vi "ExtendedKalmanFilter_New.vi"(5 "States":i32, 6 "Extended_KALMAN_FUNC_GROUP":T1, 7 "Inputs":i32, 8 "dt_Seconds":dbl=0.02, 9 "MeasurementStdDevs":T3, 10 "StateStdDevs":T3, 11 "Outputs":i32) -> (0 "Error":bool, 3 "ExtendedKalmanFiilter":T4)   [LabVIEW 2019, in "Trajectory_Library.lvlib"]
doc: "Kalman filters combine predictions from a model and measurements to give an estimate of the true system state. This is useful because many states cannot be measured directly as a result of sensor noise, or because the state is \"hidden\".\n \nThe Extended Kalman filter is just like the KalmanFilter Kalman filter, but we make a linear approximation of nonlinear dynamics and/or nonlinear measurement models. This means that the EKF works with nonlinear systems.\n\nConstructs an extended Kalman filter.\n \n - states -- the number of states.\n - inputs -- the number of inputs.\n - outputs -- the number of outputs.\n - ExtendedKalmanFuncGroup -- definition of external functions used by this filter. it includes:\n - f_func -- A vector-valued function of x and u that returns the derivative of the state vector.\n - f_FuncExtra -- extra data, if any, used by the F_Func\n - h_func -- A vector-valued function of x and u that returns the measurement vector.\n - h_FuncExtra -- extra data, if any, used by the H_Func\n - stateStdDevs -- Standard deviations of model states.\n - measurementStdDevs -- Standard deviations of measurements.\n - dtSeconds -- Nominal discretization timestep.\n\nOutputs:\n - ExtendedKalmanFilter -- filter data cluster"
uses:
  Trajectory_Library.lvlib
  <vilib>/Analysis/Matrix/Datatypes/RealMatrix.ctl
  <vilib>/Analysis/Matrix/NI_Matrix.lvlib
  TypeDef/EXTENDED_KALMAN_FILTER.ctl
  <vilib>/Analysis/NI_AALPro.lvlib
  <vilib>/Analysis/7linalg.llb/Real Transpose Matrix.vi
  TypeDef/CALLBACK_FUNC_TYPE.ctl
  TypeDef/EXTENDED_KALMAN_CORRECT_FUNC_GROUP.ctl
panel:
  # "<States,1>"
  # "<Outputs,1>"
  # "State Estimate <Statess,1>"
  # "<States, States>"
  # "<States, States>"
  # "<Statess,  States>"
  # "<Outputs, Outputs>"
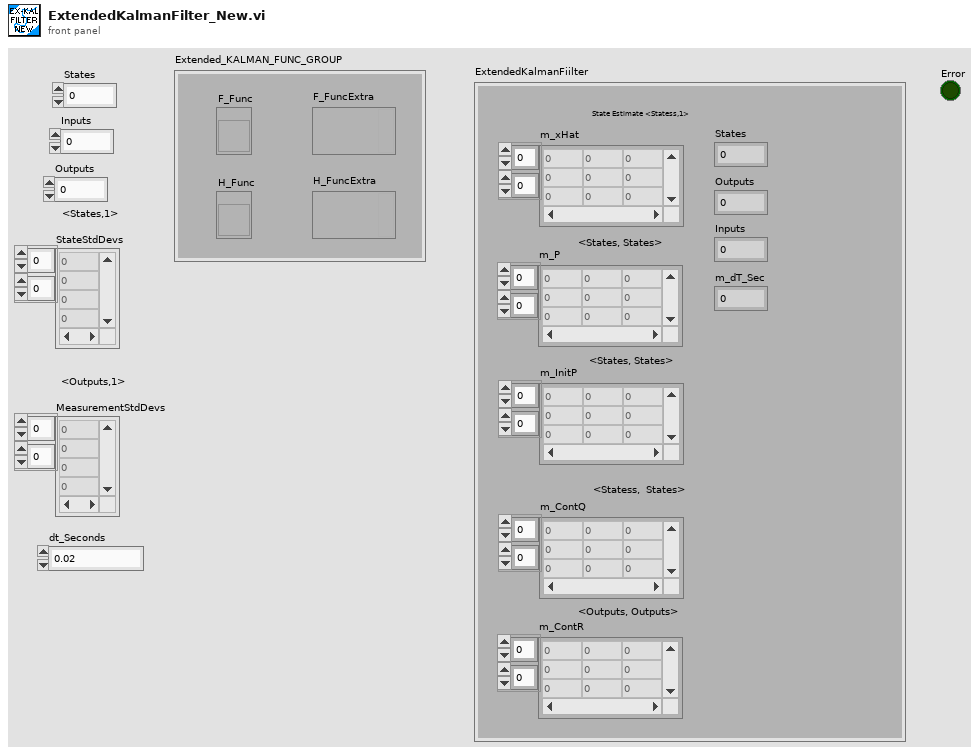
[diagram p1: front panel]
types:
  T1 = typedef "Trajectory_Library.lvlib/EXTENDED_KALMAN_CORRECT_FUNC_GROUP.ctl" = cluster{"H_Func":T2, "F_Func":T2, "H_FuncExtra":variant, "F_FuncExtra":variant}
  T2 = typedef "Trajectory_Library.lvlib/CALLBACK_FUNC_TYPE.ctl" = refnum<vi>
  T3 = typedef "NI_Matrix.lvlib/RealMatrix.ctl" = dbl[][]
  T4 = typedef "Trajectory_Library.lvlib/EXTENDED_KALMAN_FILTER.ctl" = cluster{"m_P":T3, "m_xHat":T3, "States":i32, "Outputs":i32, "m_ContR":T3, "m_ContQ":T3, "m_dT_Sec":dbl, "Inputs":i32, "m_InitP":T3}
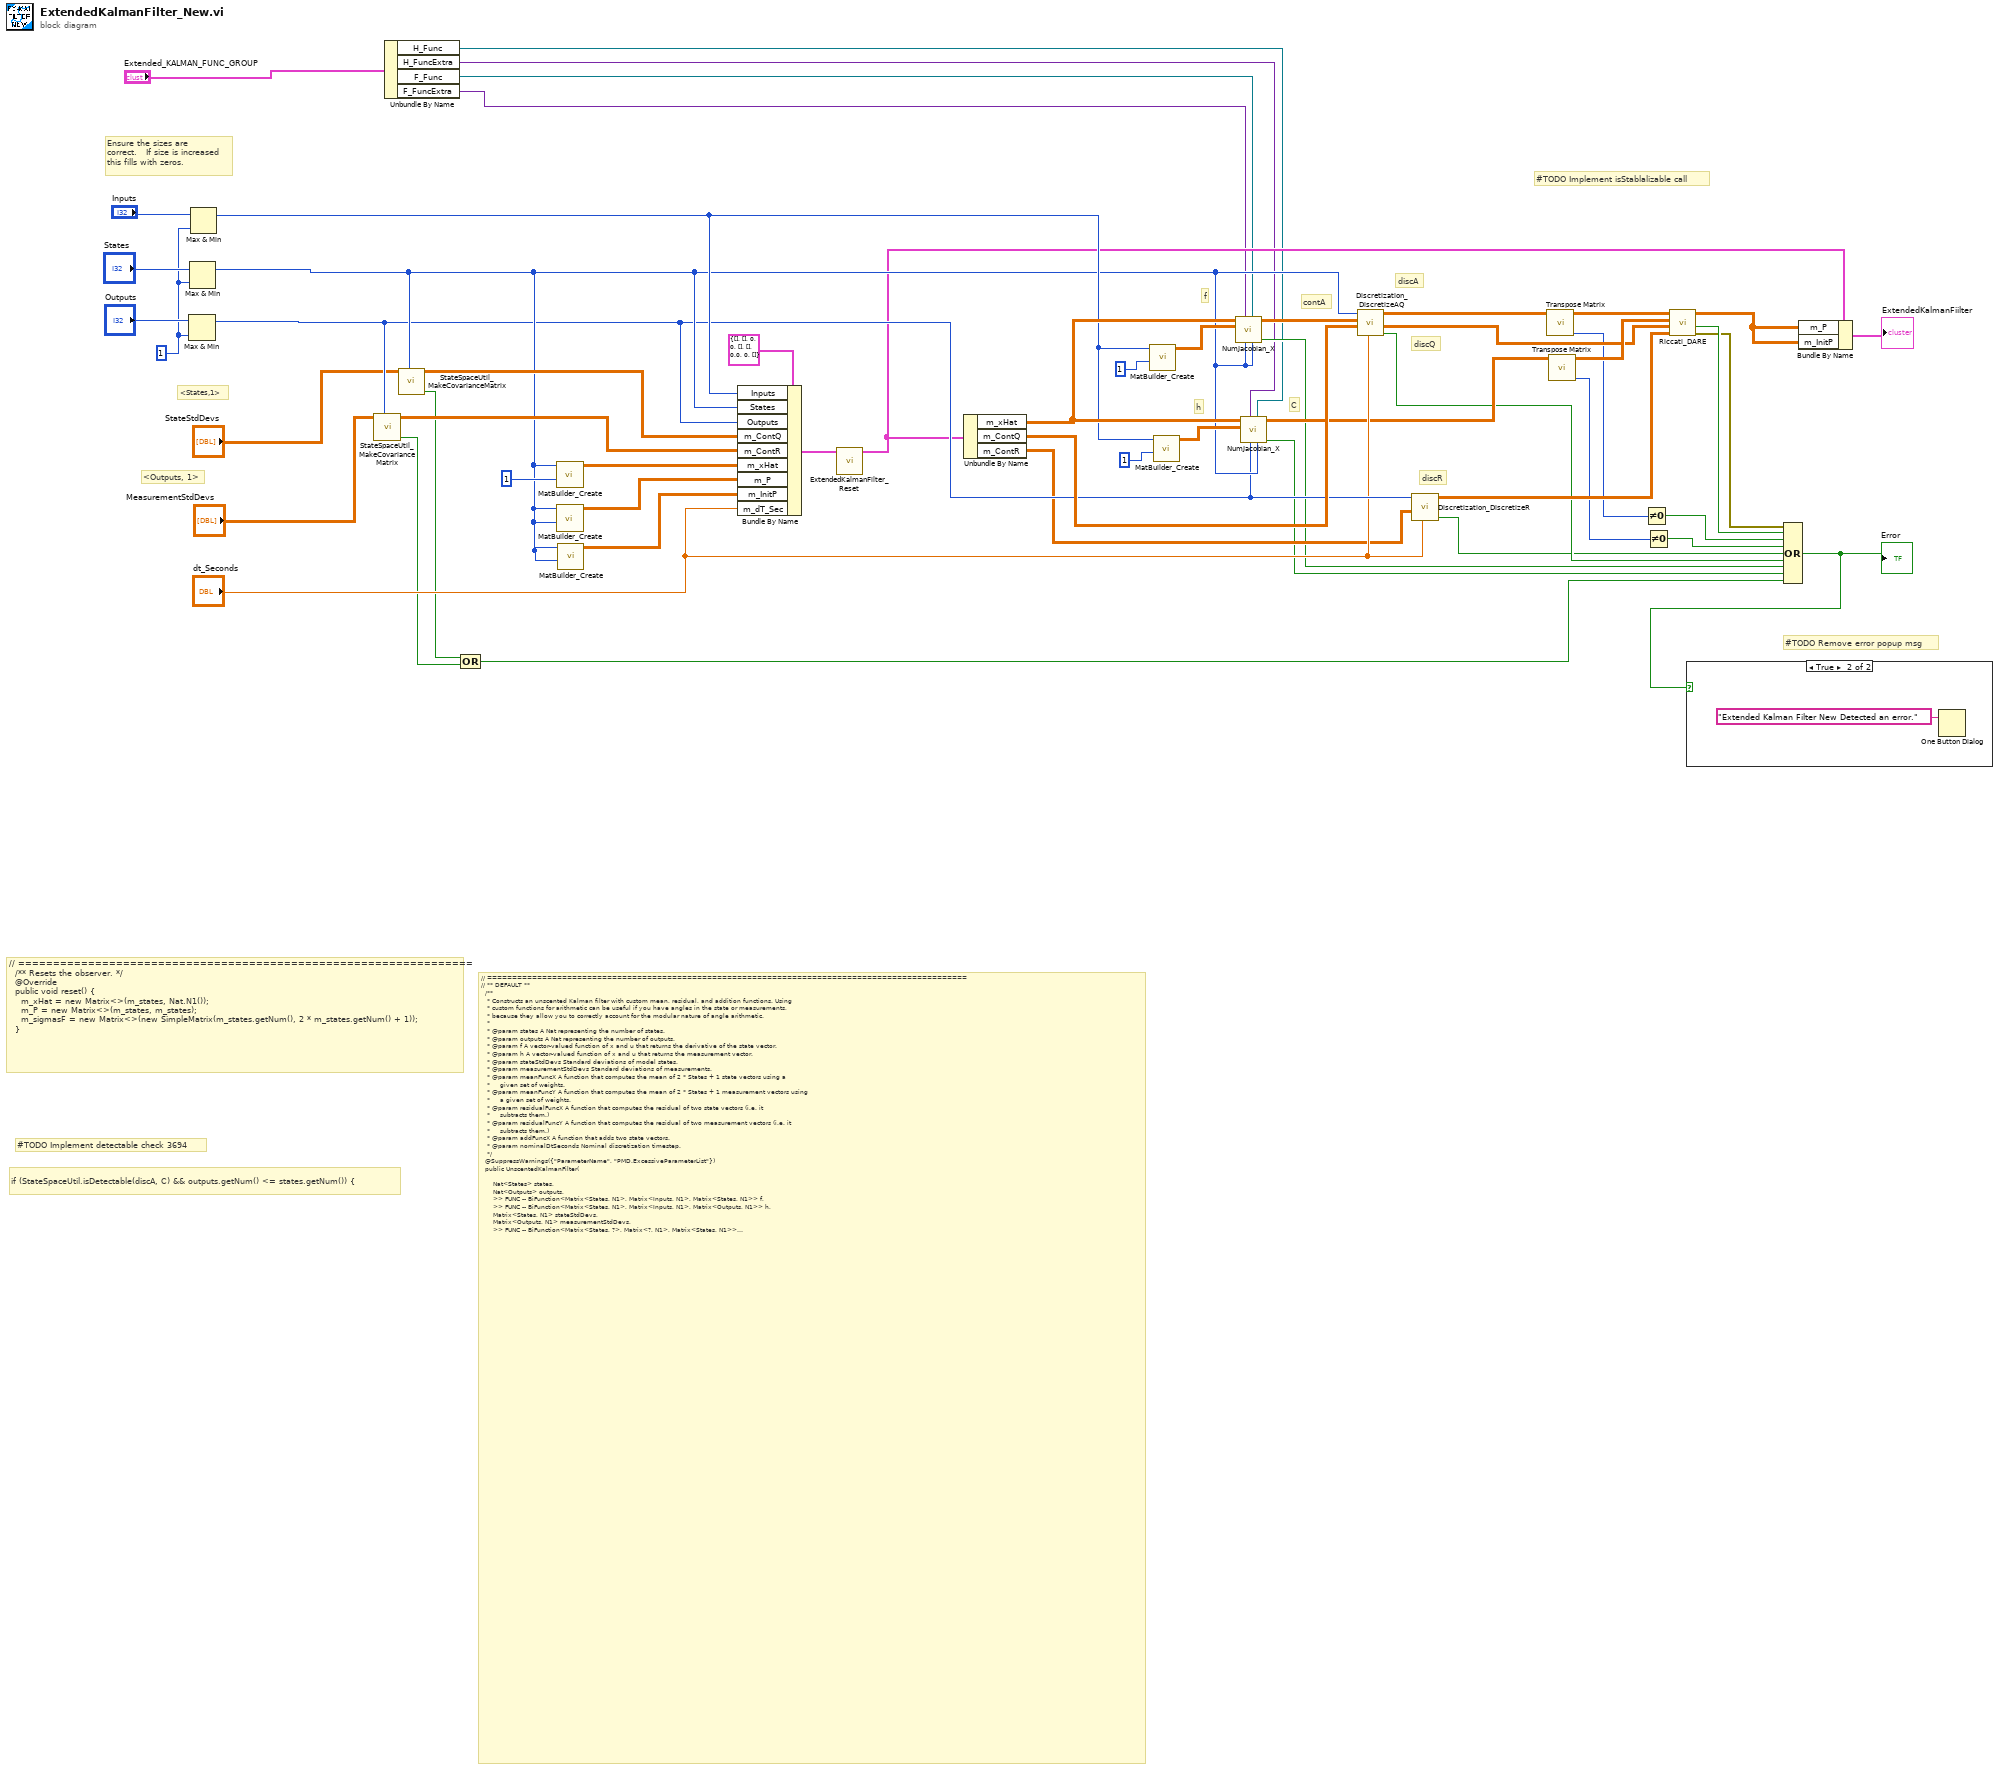
[diagram p0: block diagram]
diagram:
  w47 = 1 ("y")
  # "#TODO Implement detectable check 3694"
  # "if (StateSpaceUtil.isDetectable(discA, C) && outputs.getNum() <= states.getNum()) {"
  # "#TODO Implement isStablalizable call"
  # "discR"
  # "discQ"
  # "discA"
  # "C"
  # "contA"
  # "h"
  # "f"
  # "// =================================================================\n  /** Resets the observer. */\n  @Override\n  public void reset() {\n    m_xHat = new Matrix<>(m_states, Nat.N1());\n    m_P = new Matrix<>(m_states, m_states);\n    m_sigmasF = new Matrix<>(new SimpleMatrix(m_states.getNum(), 2 * m_states.getNum() + 1));\n  }"
  # "// ================================================================================================\n// ** DEFAULT **\n  /**\n   * Constructs an unscented Kalman filter with custom mean, residual, and addition functions. Using\n   * custom functions for arithmetic can be useful if you have angles in the state or measurements,\n   * because they allow you to correctly account for the modular nature of angle arithmetic.\n   *\n   * @param states A Nat representing the number of states.\n   * @param outputs A Nat representing the number of outputs.\n   * @param f A vector-valued function of x and u that returns the derivative of the state vector.\n   * @param h A vector-valued function of x and u that returns the measurement vector.\n   * @param stateStdDevs Standard deviations of model states.\n   * @param measurementStdDevs Standard deviations of measurements.\n   * @param meanFuncX A function that computes the mean of 2 * States + 1 state vectors using a\n   *     given set of weights.\n   * @param meanFuncY A function that computes the mean of 2 * States + 1 measurement vectors using\n   *     a given set of weights.\n   * @param residualFuncX A function that computes the residual of two state vectors (i.e. it\n   *     subtracts them.)\n   * @param residualFuncY A function that computes the residual of two measurement vectors (i.e. it\n   *     subtracts them.)\n   * @param addFuncX A function that adds two state vectors.\n   * @param nominalDtSeconds Nominal discretization timestep.\n   */\n  @SuppressWarnings({\"ParameterName\", \"PMD.ExcessiveParameterList\"})\n  public UnscentedKalmanFilter(\n\n      Nat<States> states,\n      Nat<Outputs> outputs,\n      >> FUNC -- BiFunction<Matrix<States, N1>, Matrix<Inputs, N1>, Matrix<States, N1>> f,\n      >> FUNC -- BiFunction<Matrix<States, N1>, Matrix<Inputs, N1>, Matrix<Outputs, N1>> h,\n      Matrix<States, N1> stateStdDevs,\n      Matrix<Outputs, N1> measurementStdDevs,\n      >> FUNC -- BiFunction<Matrix<States, ?>, Matrix<?, N1>, Matrix<States, N1>> meanFuncX,\n      >> FUNC -- BiFunction<Matrix<Outputs, ?>, Matrix<?, N1>, Matrix<Outputs, N1>> meanFuncY,\n      >> FUNC -- BiFunction<Matrix<States, N1>, Matrix<States, N1>, Matrix<States, N1>> residualFuncX,\n      >> FUNC -- BiFunction<Matrix<Outputs, N1>, Matrix<Outputs, N1>, Matrix<Outputs, N1>> residualFuncY,\n      >> FUNC -- BiFunction<Matrix<States, N1>, Matrix<States, N1>, Matrix<States, N1>> addFuncX,\n      double nominalDtSeconds) {\n\n    this.m_states = states;\n    this.m_outputs = outputs;\n\n    m_f = f;\n    m_h = h;\n\n    m_meanFuncX = meanFuncX;\n    m_meanFuncY = meanFuncY;\n    m_residualFuncX = residualFuncX;\n    m_residualFuncY = residualFuncY;\n    m_addFuncX = addFuncX;\n\n    m_dtSeconds = nominalDtSeconds;\n\n    m_contQ = StateSpaceUtil.makeCovarianceMatrix(states, stateStdDevs);\n    m_contR = StateSpaceUtil.makeCovarianceMatrix(outputs, measurementStdDevs);\n\n    m_pts = new MerweScaledSigmaPoints<>(states);\n\n    reset();\n  }"
  # "#TODO Remove error popup msg"
  # "<Outputs, 1>"
  # "<States,1>"
  # "Ensure the sizes are\ncorrect.   If size is increased \nthis fills with zeros."
  n1 = Max & Min(x="Outputs", y=w47) -> (max(x,y)=w33:i32)  [unwired: 1 out]
  n2 = Max & Min(x="States", y=w47) -> (max(x,y)=w34:i32)  [unwired: 1 out]
  n3 = Max & Min(x="Inputs", y=w47) -> (max(x,y)=w38:i32)  [unwired: 1 out]
  n4 = call "StateSpaceUtil_MakeCovarianceMatrix.vi"("States"=w33, "StdDevs"="MeasurementStdDevs") -> ("Size Coerced"=w6:bool, "Covariance Matrix"=w45:T3)  [unwired: 8 in]
  n5 = Unbundle By Name("Extended_KALMAN_FUNC_GROUP") -> ("H_Func"=w10:T2, "H_FuncExtra"=w11:variant, "F_Func"=w12:T2, "F_FuncExtra"=w13:variant)
  n6 = call "StateSpaceUtil_MakeCovarianceMatrix.vi"("States"=w34, "StdDevs"="StateStdDevs") -> ("Size Coerced"=w7:bool, "Covariance Matrix"=w44:T3)  [unwired: 8 in]
  n7 = Compound Arithmetic op=OR(w7, w6) -> (w16:bool)
  n8 = call "MatBuilder_Create.vi"("Columns"=1, "Rows"=w34) -> ("output matrix"=w50:T3)  [unwired: 9 in]
  n9 = call "MatBuilder_Create.vi"("Columns"=w34, "Rows"=w34) -> ("output matrix"=w49:T3)  [unwired: 9 in]
  n10 = call "MatBuilder_Create.vi"("Columns"=w34, "Rows"=w34) -> ("output matrix"=w43:T3)  [unwired: 9 in]
  n11 = Bundle By Name(cluster=T4 {"m_P"=[], "m_xHat"=[], "States"=0, "Outputs"=0, "m_ContR"=[], "m_ContQ"=[], "m_dT_Sec"=0.0, "Inputs"=0, "m_InitP"=[]} ("EXTENDED_KALMAN_FILTER"), "Inputs"=w38, "States"=w34, "Outputs"=w33, "m_ContQ"=w44, "m_ContR"=w45, "m_xHat"=w50, "m_P"=w49, "m_InitP"=w43, "m_dT_Sec"="dt_Seconds") -> (w46:T4)
  n12 = call "ExtendedKalmanFilter_Reset.vi"("in ExtendedKalmanFiilter"=w46) -> ("out ExtendedKalmanFiilter"=w24:T4)  [unwired: 10 in]
  n13 = Unbundle By Name(w24) -> ("m_xHat"=w40:T3, "m_ContQ"=w35:T3, "m_ContR"=w31:T3)
  n14 = call "MatBuilder_Create.vi"("Columns"=1, "Rows"=w38) -> ("output matrix"=w41:T3)  [unwired: 9 in]
  n15 = call "MatBuilder_Create.vi"("Columns"=1, "Rows"=w38) -> ("output matrix"=w37:T3)  [unwired: 9 in]
  n16 = call "NumJacobian_X.vi"("States"=w34, "F_FUNC"=w12, "Rows"=w34, "ExtraPassedData"=w13, "U"=w41, "X"=w40) -> ("Error"=w18:bool, "Result"=w36:T3)  [unwired: 4 in]
  n17 = call "NumJacobian_X.vi"("States"=w34, "F_FUNC"=w10, "Rows"=w33, "ExtraPassedData"=w11, "U"=w37, "X"=w40) -> ("Error"=w17:bool, "Result"=w29:T3)  [unwired: 4 in]
  n18 = call "Discretization_DiscretizeAQ.vi"("dT_Seconds"="dt_Seconds", "ContQ"=w35, "ContA"=w36, "States"=w34) -> ("Error"=w19:bool, "DiscQ"=w26:T3, "DiscA"=w30:T3)  [unwired: 5 in]
  n19 = call "Discretization_DiscretizeR.vi"("dT_Seconds"="dt_Seconds", "ContR"=w31, "Outputs"=w33) -> ("Size Coerced"=w2:bool, "DiscR"=w25:T3)  [unwired: 7 in]
  n20 = call-poly <vilib>:"Transpose Matrix.vi"("Input Matrix"=w30) -> ("error"=w21:i32, "Matrix Transpose"=w28:T3)  [unwired: 9 in]
  n21 = call-poly <vilib>:"Transpose Matrix.vi"("Input Matrix"=w29) -> ("error"=w20:i32, "Matrix Transpose"=w27:T3)  [unwired: 9 in]
  n22 = Not Equal To 0?(x=w21) -> (x != 0?=w4:bool)
  n23 = Not Equal To 0?(x=w20) -> (x != 0?=w3:bool)
  n24 = call "Riccati_DARE.vi"("R"=w25, "Q"=w26, "B"=w27, "A"=w28) -> ("error out"=w1:errorcluster, "Error"=w5:bool, "Answer"=w23:T3)  [unwired: 4 in, 1 out]
  n25 = Compound Arithmetic op=OR(w1, w5, w4, w3, w2, w19, w18, w17, w16) -> (w15:bool)
  "Error" <- w15
  n26 = case shown="True" w15 {
    frame False {
    }
    frame True {
      n27 = One Button Dialog(message="Extended Kalman Filter New Detected an error.") -> ()  [unwired: 1 in, 1 out]
    }
  }
  n28 = Bundle By Name(cluster=w24, "m_P"=w23, "m_InitP"=w23) -> (→"ExtendedKalmanFiilter":T4)
